vi "Prepare Input Buffer.vi"(11 "String to Encode":string) -> (3 "Chunked MEssage":u8[][](array[numeric]) format="%02x")   [LabVIEW 2018, in "SHA256.lvlib"]
doc: "Takes a message for SHA-256 hashing and converts it in 512 bit chunks, padding with zeros as necessary and including the length a terminating bit."
uses:
  SHA256.lvlib
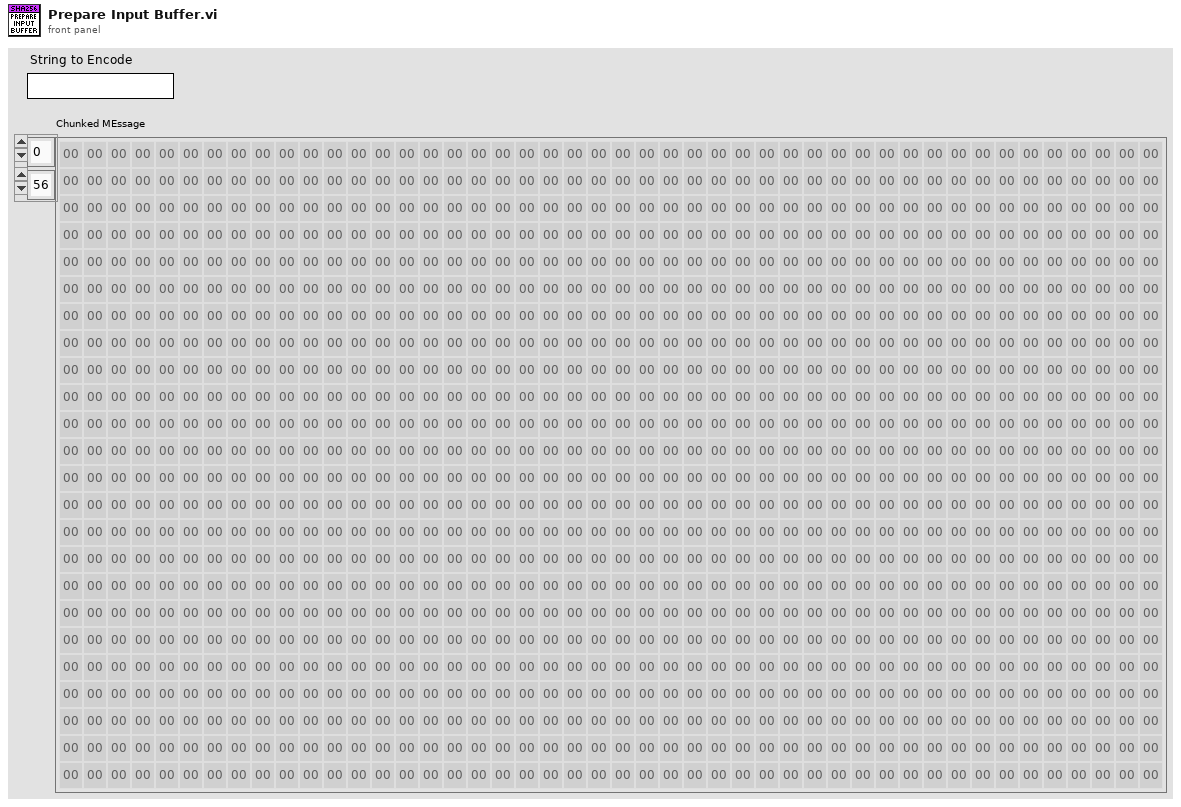
[diagram p1: front panel]
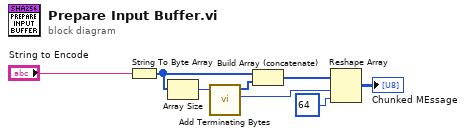
[diagram p0: block diagram]
diagram:
  n1 = String To Byte Array(string="String to Encode") -> (unsigned byte array=w4:u8[])
  n2 = Array Size(array=w4) -> (size(s)=w2:i32)
  n3 = call "Add Terminating Bytes.vi"("Size of Data"=w2) -> ("Number of Chunks"=w7:i32, "Array"=w3:u8[])  [unwired: 8 in, 1 out]
  n4 = Build Array (concatenate)(w4, w3) -> (w1:u8[])
  n5 = Reshape Array(w1, w7, 64 ("dimension size")) -> (→"Chunked MEssage":u8[][])
